vi "Source V1.vi"(8 "error in":errorcluster, 9 "V1 rate":dbl, 10 "V1":dbl, 11 "VISA in":refnum<visa-resource-name>) -> (0 "error out":errorcluster, 1 "read buffer":string, 2 "format string":string="SOUR1:VOLT %3f.4:SLEW %3f.4", 3 "VISA out":refnum<visa-resource-name>)   [LabVIEW 2016, in "RP100.lvclass"]
uses:
  RP100.lvclass
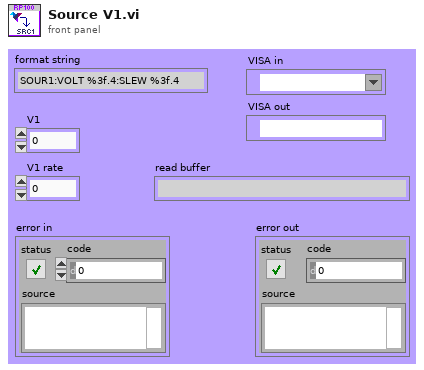
[diagram p1: front panel]
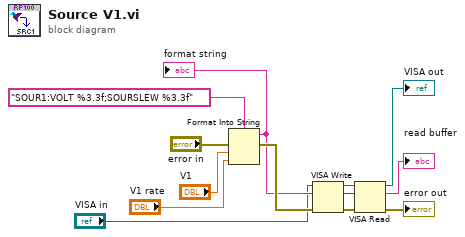
[diagram p0: block diagram]
diagram:
  n1 = Format Into String(format string="SOUR1:VOLT %3.3f;SOURSLEW %3.3f", error in="error in", "V1", "V1 rate") -> (resulting string=w9:string, error out=w11:errorcluster)  [unwired: 1 in]
  "format string" <- w9
  n2 = VISA Write(VISA resource name="VISA in", write buffer=w9, error in (no error)=w11) -> (VISA resource name out=w6:refnum<visa-resource-name>, return count=w5:u32, error out=w3:errorcluster)
  n3 = VISA Read(VISA resource name=w6, byte count=w5, error in (no error)=w3) -> (VISA resource name out=→"VISA out":refnum<visa-resource-name>, read buffer=→"read buffer":string, error out=→"error out":errorcluster)  [unwired: 1 out]
